vi "Sensors Global.vi"() -> ()   [LabVIEW 2014, in "Elevator System.lvlib"]
uses:
  Elevator System.lvlib
panel:
  in  "Gripper Sensor R":dbl
  in  "Gripper Sensor L":dbl
  in  "Elevator Sensor":dbl
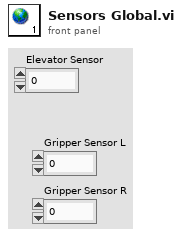
[diagram p1: front panel]
diagram:
